vi "Reconnect.vi"(8 "error in (no error)":errorcluster, 11 "TwinCAT ADS in":refnum<class "TwinCAT ADS.lvclass">) -> (0 "error out":errorcluster, 3 "TwinCAT ADS out":refnum<class "TwinCAT ADS.lvclass">)   [LabVIEW 2018, in "TwinCAT ADS.lvclass"]
uses:
  TwinCAT ADS.lvclass
  TwinCAT ADS.lvclass/TwinCAT ADS.ctl
  TwinCAT.Ads
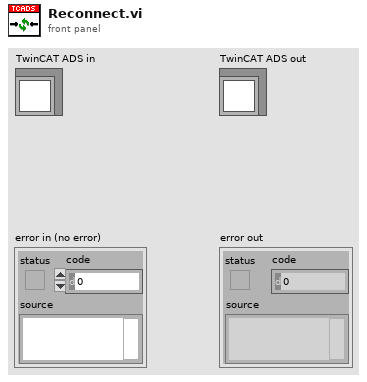
[diagram p1: front panel]
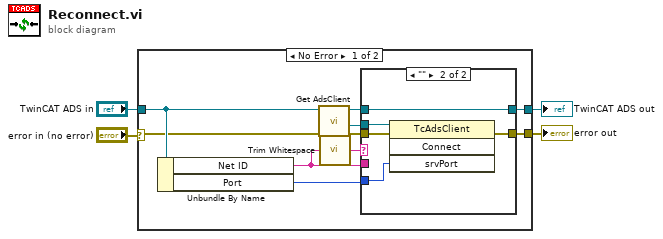
[diagram p0: block diagram]
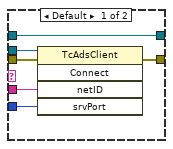
[diagram p2: hidden frame]
diagram:
  n1 = case shown="No Error" "error in (no error)" {
    selector: "error in (no error)" -> [w7 w27]
    tunnel: [w5 w27] -> w3
    tunnel: [w6 w26] -> w1
    tunnel: "TwinCAT ADS in" -> [w13 w26]
    frame No Error {
      n2 = Unbundle By Name(w13) -> ("Net ID"=w9:string, "Port"=w12:i32)
      n3 = call "Get AdsClient.vi"("error in (no error)"=w7, "TwinCAT ADS in"=w13) -> ("error out"=w14:errorcluster, ".NET TcAdsClient"=w10:refnum<k24>, "TwinCAT ADS out"=w8:refnum<class "TwinCAT ADS.lvclass">)  [unwired: 7 in]
      n4 = call <vilib>:"Trim Whitespace.vi"("string"=w9) -> ("trimmed string"=w11:string)  [unwired: 1 in]
      n5 = case shown="\"\"" w11 {
        tunnel: w14 -> [w20 w25]
        tunnel: w12 -> [w19 w22]
        tunnel: w10 -> [w18 w24]
        tunnel: [w17 w23] -> w5
        tunnel: w9 -> [w16 _]
        tunnel: w8 -> [w15 w21]
        tunnel: [w15 w21] -> w6
        frame Default {
          n6 = invoke class="TcAdsClient" method="Connect"(reference=w18, error in=w20, "netID"=w16, "srvPort"=w19) -> (error out=w17:errorcluster)  [unwired: 1 in, 4 out]
        }
        frame "" {
          n7 = invoke class="TcAdsClient" method="Connect"(reference=w24, error in=w25, "srvPort"=w22) -> (error out=w23:errorcluster)  [unwired: 1 in, 3 out]
        }
      }
    }
    frame Error {
    }
  }
  "error out" <- w3
  "TwinCAT ADS out" <- w1
